vi "Decode Type Descriptor.vi"(4 "error in (no error)":errorcluster, 7 "TypeDesc":i16[](array[numeric])) -> (0 "error out":errorcluster, 1 "Type Descriptor":i16[](array[numeric]), 2 "Control Label":string, 3 "Type String":string)   [LabVIEW 2010]
doc: "In decoding the type descriptor, data types that contain other data types need to be handled differently. Specifically, these would be arrays and clusters. The generic term \"blob\" is used throughout this program to refer to these types as a whole.\n\nThe string output by this code is generally not useful to send to another VI, but it is obvious how it corresponds to the data type of the input. The purpose of the code is to see how the type descriptor is formatted and how to decode it.\n\nThe low byte of the appropriate element of the type descriptor array contains the type of the data. See small string selection case and large operate case for what data types correspond to what numbers.\n\nThe blob parameter arrays in the shift registers (size, index, element, done, dimension) are manipulated as a stack to allow decoding even deeply nested data types.\n\nGenerally, each case in the large operate case structure performs the following tasks:\n1. Uses \"Calculate String Info.vi\" and \"Replace Substring\" to assemble the type string.\n2. Uses \"Calculate Blob Info.vi\" to calculate the next type descriptor index position.\n3. Parses out the label for the control in question from the type descriptor array.\n\nThis VI is complicated in order to support nested data types such as a cluster of arrays of clusters. For more information on the format of the type descriptor, see app note 154 at ni.com, entitled \"LabVIEW Data Storage\"."
panel:
  # "Select Help»Show Context Help and move the cursor\nover the VI icon to display help for this VI."
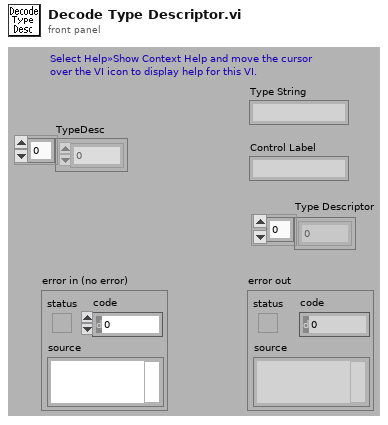
[diagram p1: front panel]
types:
  T1 = cluster{"status":bool, "code":i32, "name":string}
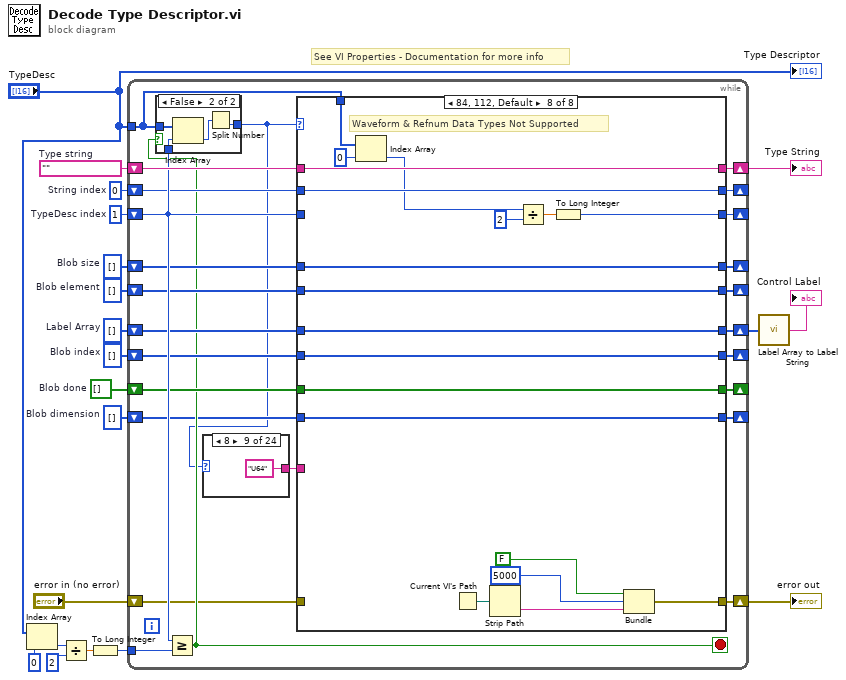
[diagram p0: block diagram]
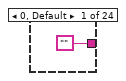
[diagram p2: hidden frame]
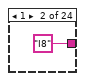
[diagram p3: hidden frame]
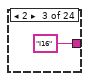
[diagram p4: hidden frame]
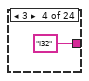
[diagram p5: hidden frame]
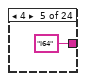
[diagram p6: hidden frame]
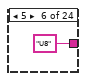
[diagram p7: hidden frame]
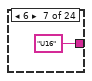
[diagram p8: hidden frame]
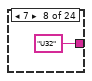
[diagram p9: hidden frame]
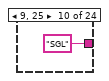
[diagram p10: hidden frame]
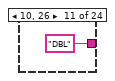
[diagram p11: hidden frame]
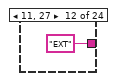
[diagram p12: hidden frame]
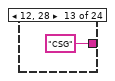
[diagram p13: hidden frame]
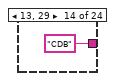
[diagram p14: hidden frame]
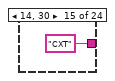
[diagram p15: hidden frame]
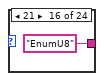
[diagram p16: hidden frame]
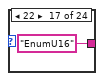
[diagram p17: hidden frame]
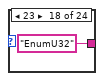
[diagram p18: hidden frame]
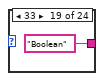
[diagram p19: hidden frame]
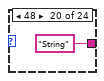
[diagram p20: hidden frame]
diagram:
  w2 = i16[] []  # Blob dimension
  w5 = i16[] []  # Blob index
  w6 = bool[] []  # Blob done
  w7 = i16[] []  # Blob element
  w8 = i16[] []  # Blob size
  w10 = i16[] []  # Label Array
  w11 = 0  # String index
  w14 = 1  # TypeDesc index
  w20 = ""  # Type string
  # "See VI Properties - Documentation for more info"
  n1 = Index Array(array="TypeDesc", index=0) -> (element=w18:i16)
  n2 = Divide(x=w18, y=i16 2) -> (x/y=w16:dbl)
  n3 = To Long Integer(number=w16) -> (32bit integer=w15:i32)
  n4 = while {
    shift-left: w2 -> [w23]
    shift-right: [w22] -> _
    shift-left: "error in (no error)" -> [w25]
    shift-right: [w24] -> w4
    shift-left: w5 -> [w30]
    shift-right: [w29] -> _
    shift-left: w6 -> [w32]
    shift-right: [w31] -> _
    shift-left: w10 -> [w34]
    shift-right: [w35] -> w9
    shift-left: w7 -> [w37]
    shift-right: [w36] -> _
    shift-left: w8 -> [w39]
    shift-right: [w38] -> _
    shift-left: w11 -> [w41]
    shift-right: [w40] -> _
    shift-left: w14 -> [w42]
    shift-right: [w45] -> _
    tunnel: w15 -> [w27]
    shift-left: w20 -> [w44]
    shift-right: [w43] -> w12
    tunnel: "TypeDesc" -> [w33]
    stop <- w28 stop-if-true
    n5 = Greater Or Equal?(x=w42, y=w27) -> (x >= y?=w28:bool)
    n6 = case shown="False" w28 {
      tunnel: w33 -> [_ w74]
      tunnel: [u8 0 w72] -> w21
      tunnel: w42 -> [_ w71]
      frame True {
      }
      frame False {
        n7 = Index Array(array=w74, index=w71) -> (element=w73:i16)
        n8 = Split Number(x=w73) -> (lo(x)=w72:u8)  [unwired: 1 out]
      }
    }
    n9 = case shown="8" w21 {
      tunnel: ["" "I8" ("string") "I16" ("string") "I32" ("string") "I64" ("string") "U8" ("string") "U16" ("string") "U32" ("string") "U64" ("string") "SGL" ("string") "DBL" ("string") "EXT" ("string") "CSG" ("string") "CDB" ("string") "CXT" ("string") "EnumU8" ("string") "EnumU16" ("string") "EnumU32" ("string") "Boolean" ("string") "String" ("string") "Path" ("string") "Pict" ("string") "ArrayD()" ("string") "Cluster()" ("string")] -> w26
      frame 0, Default {
      }
      frame 1 {
      }
      frame 2 {
      }
      frame 3 {
      }
      frame 4 {
      }
      frame 5 {
      }
      frame 6 {
      }
      frame 7 {
      }
      frame 8 {
      }
      frame 9, 25 {
      }
      frame 10, 26 {
      }
      frame 11, 27 {
      }
      frame 12, 28 {
      }
      frame 13, 29 {
      }
      frame 14, 30 {
      }
      frame 21 {
      }
      frame 22 {
      }
      frame 23 {
      }
      frame 33 {
      }
      frame 48 {
      }
      frame 50 {
      }
      frame 51 {
      }
      frame 64 {
      }
      frame 80 {
      }
    }
    n10 = case shown="84, 112, Default" w21 {
      tunnel: [w77 w97 w140 w186 w217 w247 w358 w450] -> w45
      tunnel: w42 -> [w77 w89 w130 w176 w209 w252 w363 _]
      tunnel: [w84 w106 w148 w195 w226 w255 w366 w462] -> w43
      tunnel: w44 -> [w84 w107 w149 w196 w227 w256 w367 w462]
      tunnel: [w80 w108 w116 w197 w228 w243 w354 w458] -> w35
      tunnel: w41 -> [w83 w95 w138 w184 w215 w254 w365 w461]
      tunnel: [w83 w91 w134 w180 w211 w253 w364 w461] -> w40
      tunnel: [w82 w101 w143 w190 w221 w248 w359 w460] -> w38
      tunnel: w39 -> [w82 w94 w137 w183 w214 w251 w362 w460]
      tunnel: [w81 w102 w144 w191 w222 w249 w360 w459] -> w36
      tunnel: w37 -> [w81 w93 w136 w182 w213 w250 w361 w459]
      tunnel: w34 -> [w80 _ _ _ _ _ _ w458]
      tunnel: w33 -> [_ w90 w121 w177 w210 w239 w350 w455]
      tunnel: w32 -> [w79 w104 w146 w193 w224 w242 w353 w456]
      tunnel: [w79 w103 w145 w192 w223 w246 w357 w456] -> w31
      tunnel: w30 -> [w78 w99 w142 w188 w219 w245 w356 w457]
      tunnel: [w78 w98 w141 w187 w218 w244 w355 w457] -> w29
      tunnel: w26 -> [_ w87 w132 w179 w207 w238 w349 _]
      tunnel: w25 -> [w76 w86 w131 w178 w204 w237 w348 _]
      tunnel: [w76 w86 w131 w178 w204 w237 w348 w445] -> w24
      tunnel: [w75 w85 w115 w167 w203 w235 w346 w444] -> w22
      tunnel: w23 -> [w75 w85 w115 w167 w203 w236 w347 w444]
      frame 0 {
        # "No-op, finished"
      }
      frame 1..14, 33 {
        # "Scalar Numeric & Boolean Data Types"
        n11 = Decrement(x=w89) -> (x-1=w88:i32)
        n12 = call "Calculate String Info.vi"("Str in"=w87, "Str idx in"=w95, "Blob size in"=w94, "Blob elem in"=w93, "Is scalar"=TRUE) -> ("Str out"=w92:string, "Str idx out"=w91:i32)  [unwired: 9 out]
        n13 = Index Array(array=w90, index=w88) -> (element=w100:i16)
        n14 = call "Calculate Blob Info.vi"("TypeDesc idx in"=w89, "Sub-desc size"=w100, "Blob size in"=w94, "Blob elem in"=w93, "Blob idx in"=w99, "Blob done in"=w104, "Blob dim"=w85) -> ("TypeDesc idx out"=w97:i32, "Blob size out"=w101:i16[], "Blob elem out"=w102:i16[], "Blob idx out"=w98:i16[], "Blob done out"=w103:bool[])  [unwired: 4 out]
        n15 = Divide(x=w100, y=i16 2) -> (x/y=w113:dbl)
        n16 = Replace Substring(2:0 ("length (len. of substring)"), 3:w95, 4:w92, 5:w107) -> (1:w106:string)  [unwired: 1 out]
        n17 = To Long Integer(number=w113) -> (32bit integer=w112:i32)
        n18 = Increment(x=w89) -> (x+1=w114:i32)
        n19 = Subtract(x=w112, y=2) -> (x-y=w109:i32)
        n20 = Array Subset(array=w90, index=w114, length=w109) -> (w108:i16[])
      }
      frame 21..23 {
        # "Enumerated Integer Data Types"
        n21 = Increment(x=w130) -> (x+1=w127:i32)
        n22 = Decrement(x=w130) -> (x-1=w133:i32)
        n23 = call "Calculate String Info.vi"("Str in"=w132, "Str idx in"=w138, "Blob size in"=w137, "Blob elem in"=w136, "Is scalar"=TRUE) -> ("Str out"=w135:string, "Str idx out"=w134:i32)  [unwired: 9 out]
        n24 = Index Array(array=w121, index=w133) -> (element=w120:i16)
        n25 = Index Array(array=w121, index=w127) -> (element=w129:i16)
        n26 = Increment(x=w127) -> (x+1=w126:i32)
        n27 = call "Calculate Blob Info.vi"("TypeDesc idx in"=w130, "Sub-desc size"=w120, "Blob size in"=w137, "Blob elem in"=w136, "Blob idx in"=w142, "Blob done in"=w146, "Blob dim"=w115) -> ("TypeDesc idx out"=w140:i32, "Blob size out"=w143:i16[], "Blob elem out"=w144:i16[], "Blob idx out"=w141:i16[], "Blob done out"=w145:bool[])  [unwired: 4 out]
        n28 = To Long Integer(number=w129) -> (32bit integer=w128:i32)
        n29 = for {
          N: w128 -> [_]
          shift-right: [w150] -> w123
          shift-left: w126 -> [w155]
          tunnel: w121 -> [w166]
          shift-right: [w159] -> w124
          shift-left: TRUE -> [w156]
          n30 = Index Array(array=w166, index=w155) -> (element=w165:i16)
          n31 = Split Number(x=w165) -> (hi(x)=w164:u8, lo(x)=w163:u8)
          n32 = Select(t=w164, s=w156, f=w163) -> (s? t:f=w158:u8)
          n33 = Quotient & Remainder(x=w158, y=u8 2) -> (x-y*floor(x/y)=w161:u8, floor(x/y)=w160:u8)
          n34 = To Long Integer(number=w160) -> (32bit integer=w154:i32)
          n35 = Equal To 0?(x=w161) -> (x = 0?=w157:bool)
          n36 = And(x=w156, y=w157) -> (x .and. y?=w153:bool)
          n37 = Add(x=w154, y=w155) -> (x+y=w152:i32)
          n38 = Increment(x=w152) -> (x+1=w151:i32)
          n39 = Exclusive Or(1:w156, 2:w157) -> (0:w159:bool)
          n40 = Select(t=w152, s=w153, f=w151) -> (s? t:f=w150:i32)
        }
        n41 = Increment(x=w123) -> (x+1=w122:i32)
        n42 = To Long Integer(number=w120) -> (32bit integer=w118:i32)
        n43 = Select(t=w123, s=w124, f=w122) -> (s? t:f=w119:i32)
        n44 = Subtract(x=w118, y=w119) -> (x-y=w117:i32)
        n45 = Array Subset(array=w121, index=w119, length=w117) -> (w116:i16[])
        n46 = Replace Substring(2:0 ("length (len. of substring)"), 3:w138, 4:w135, 5:w149) -> (1:w148:string)  [unwired: 1 out]
      }
      frame 25..30 {
        # "Physical Quantity Scalar Numeric Data Types"
        n47 = Decrement(x=w176) -> (x-1=w169:i32)
        n48 = call "Calculate String Info.vi"("Str in"=w179, "Str idx in"=w184, "Blob size in"=w183, "Blob elem in"=w182, "Is scalar"=TRUE) -> ("Str out"=w181:string, "Str idx out"=w180:i32)  [unwired: 9 out]
        n49 = Increment(x=w176) -> (x+1=w175:i32)
        n50 = Index Array(array=w177, index=w175) -> (element=w174:i16)
        n51 = Index Array(array=w177, index=w169) -> (element=w189:i16)
        n52 = call "Calculate Blob Info.vi"("TypeDesc idx in"=w176, "Sub-desc size"=w189, "Blob size in"=w183, "Blob elem in"=w182, "Blob idx in"=w188, "Blob done in"=w193, "Blob dim"=w167) -> ("TypeDesc idx out"=w186:i32, "Blob size out"=w190:i16[], "Blob elem out"=w191:i16[], "Blob idx out"=w187:i16[], "Blob done out"=w192:bool[])  [unwired: 4 out]
        n53 = Multiply(x=w174, y=i16 2) -> (x*y=w172:i16)
        n54 = Divide(x=w189, y=i16 2) -> (x/y=w201:dbl)
        n55 = Add(x=w172, y=i16 3) -> (x+y=w170:i16)
        n56 = Replace Substring(2:0 ("length (len. of substring)"), 3:w184, 4:w181, 5:w196) -> (1:w195:string)  [unwired: 1 out]
        n57 = To Long Integer(number=w201) -> (32bit integer=w200:i32)
        n58 = To Long Integer(number=w170) -> (32bit integer=w168:i32)
        n59 = Add(x=w168, y=w169) -> (x+y=w202:i32)
        n60 = Subtract(x=w200, y=w168) -> (x-y=w198:i32)
        n61 = Array Subset(array=w177, index=w202, length=w198) -> (w197:i16[])
      }
      frame 48, 50, 51 {
        # "String, Path, & Pict Data Types"
        n62 = Decrement(x=w209) -> (x-1=w208:i32)
        n63 = call "Calculate String Info.vi"("Str in"=w207, "Str idx in"=w215, "Blob size in"=w214, "Blob elem in"=w213, "Is scalar"=TRUE) -> ("Str out"=w212:string, "Str idx out"=w211:i32)  [unwired: 9 out]
        n64 = Index Array(array=w210, index=w208) -> (element=w220:i16)
        n65 = call "Calculate Blob Info.vi"("TypeDesc idx in"=w209, "Sub-desc size"=w220, "Blob size in"=w214, "Blob elem in"=w213, "Blob idx in"=w219, "Blob done in"=w224, "Blob dim"=w203) -> ("TypeDesc idx out"=w217:i32, "Blob size out"=w221:i16[], "Blob elem out"=w222:i16[], "Blob idx out"=w218:i16[], "Blob done out"=w223:bool[])  [unwired: 4 out]
        n66 = Divide(x=w220, y=i16 2) -> (x/y=w233:dbl)
        n67 = Increment(x=w209) -> (x+1=w205:i32)
        n68 = Replace Substring(2:0 ("length (len. of substring)"), 3:w215, 4:w212, 5:w227) -> (1:w226:string)  [unwired: 1 out]
        n69 = To Long Integer(number=w233) -> (32bit integer=w232:i32)
        n70 = Increment(x=w205) -> (x+1=w206:i32)
        n71 = Increment(x=w206) -> (x+1=w234:i32)
        n72 = Subtract(x=w232, y=4) -> (x-y=w229:i32)
        n73 = Array Subset(array=w210, index=w234, length=w229) -> (w228:i16[])
      }
      frame 64 {
        # "Array"
        n74 = Index Array(array=w242, index=0) -> (element=w240:bool)
        n75 = case shown="True" w240 {
          tunnel: w256 -> [w293 w342]
          tunnel: [w292 w342] -> w255
          tunnel: w254 -> [w274 w314]
          tunnel: [w277 w317] -> w253
          tunnel: w252 -> [w290 w306]
          tunnel: w251 -> [w273 w313]
          tunnel: w250 -> [w272 w340]
          tunnel: [w289 w320] -> w249
          tunnel: [w288 w321] -> w248
          tunnel: [w266 w325] -> w247
          tunnel: w242 -> [w285 w341]
          tunnel: [w283 w318] -> w246
          tunnel: w245 -> [w281 w337]
          tunnel: [w280 w319] -> w244
          tunnel: [i16[] [] w334] -> w243
          tunnel: w239 -> [w275 w310]
          tunnel: w238 -> [w263 _]
          tunnel: w236 -> [w259 w297]
          tunnel: [w258 w307] -> w235
          frame False {
            w271 = i16 1 ("new element/subarray")
            w260 = 0 ("index")
            n76 = Increment(x=w290) -> (x+1=w287:i32)
            n77 = Index Array(array=w275, index=w287) -> (element=w257:i16)
            n78 = Number To Decimal String(number=w257) -> (decimal integer string=w261:string)  [unwired: 1 out]
            n79 = Increment(x=w287) -> (x+1=w286:i32)
            n80 = Multiply(x=w257, y=i16 2) -> (x*y=w268:i16)
            n81 = Increment(x=w286) -> (x+1=w269:i32)
            n82 = To Long Integer(number=w268) -> (32bit integer=w267:i32)
            n83 = Insert Into Array(array=w273, index=w260, new element=w271) -> (w288:i16[])
            n84 = Insert Into Array(array=w272, index=w260, new element=w271) -> (w289:i16[])
            n85 = Insert Into Array(array=w281, index=w260, new element=i16 0) -> (w280:i16[])
            n86 = Insert Into Array(array=w285, index=w260, new element=FALSE ("new element/subarray")) -> (w283:bool[])
            n87 = Insert Into Array(array=w259, index=w260, new element=w257) -> (w258:i16[])
            n88 = Replace Substring(2:0 ("length (len. of substring)"), 3:5 ("offset (0)"), 4:w261, 5:w263) -> (1:w262:string)  [unwired: 1 out]
            n89 = Add(x=w267, y=w269) -> (x+y=w266:i32)
            n90 = call "Calculate String Info.vi"("Str in"=w262, "Str idx in"=w274, "Blob size in"=w273, "Blob elem in"=w272, "Is scalar"=FALSE) -> ("Str out"=w278:string, "Str idx out"=w277:i32)  [unwired: 9 out]
            n91 = Replace Substring(2:0 ("length (len. of substring)"), 3:w274, 4:w278, 5:w293) -> (1:w292:string)  [unwired: 1 out]
          }
          frame True {
            w339 = 0 ("index")
            w338 = 1 ("length")
            n92 = Decrement(x=w306) -> (x-1=w311:i32)
            n93 = Index Array(array=w310, index=w311) -> (element=w309:i16)
            n94 = Index Array(array=w337, index=0) -> (element=w329:i16)
            n95 = Delete From Array(array=w313, length=w338, index=w339) -> (array with subset deleted=w312:i16[])  [unwired: 1 out]
            n96 = Delete From Array(array=w340, length=w338, index=w339) -> (array with subset deleted=w324:i16[])  [unwired: 1 out]
            n97 = Delete From Array(array=w337, length=w338, index=w339) -> (array with subset deleted=w323:i16[])  [unwired: 1 out]
            n98 = Delete From Array(array=w341, length=w338, index=w339) -> (array with subset deleted=w322:bool[])  [unwired: 1 out]
            n99 = Subtract(x=w309, y=w329) -> (x-y=w332:i16)
            n100 = Divide(x=w329, y=i16 2) -> (x/y=w328:dbl)
            n101 = Array Size(array=w312) -> (size(s)=w316:i32)
            n102 = Divide(x=w332, y=i16 2) -> (x/y=w333:dbl)
            n103 = To Long Integer(number=w328) -> (32bit integer=w327:i32)
            n104 = Delete From Array(array=w297, length=1 ("index"), index=0 ("length")) -> (array with subset deleted=w307:i16[])  [unwired: 1 out]
            n105 = call "Calculate Blob Info.vi"("TypeDesc idx in"=w306, "Sub-desc size"=w309, "Blob size in"=w312, "Blob elem in"=w324, "Blob idx in"=w323, "Blob done in"=w322, "Blob dim"=w307) -> ("TypeDesc idx out"=w325:i32, "Blob size out"=w321:i16[], "Blob elem out"=w320:i16[], "Blob idx out"=w319:i16[], "Blob done out"=w318:bool[])  [unwired: 4 out]
            n106 = To Long Integer(number=w333) -> (32bit integer=w302:i32)
            n107 = Not Equal To 0?(x=w316) -> (x != 0?=w315:bool)
            n108 = Add(x=w327, y=2) -> (x+y=w305:i32)
            n109 = Index Array(array=w297, index=0) -> (element=w295:i16)
            n110 = case shown="True" w315 {
              tunnel: w314 -> [w343 w345]
              tunnel: [w343 w344] -> w317
              frame False {
              }
              frame True {
                n111 = Increment(x=w345) -> (x+1=w344:i32)
              }
            }
            n112 = To Long Integer(number=w295) -> (32bit integer=w300:i32)
            n113 = Multiply(x=w300, y=2) -> (x*y=w294:i32)
            n114 = Compound Arithmetic op=ADD(w306, w305, w294) -> (w304:i32)
            n115 = Compound Arithmetic op=ADD(w305, w294, 3 ("y")) -> (w301:i32)
            n116 = Subtract(x=w301, y=w302) -> (x-y=w331:i32)
            n117 = Array Subset(array=w310, index=w304, length=w331) -> (w334:i16[])
          }
        }
      }
      frame 80 {
        # "Cluster"
        n118 = Index Array(array=w353, index=0) -> (element=w351:bool)
        n119 = case shown="True" w351 {
          tunnel: w367 -> [w397 w440]
          tunnel: [w396 w440] -> w366
          tunnel: w365 -> [w376 w408]
          tunnel: [w379 w411] -> w364
          tunnel: w363 -> [w394 w398]
          tunnel: w362 -> [w375 w407]
          tunnel: w361 -> [w374 w438]
          tunnel: [w391 w414] -> w360
          tunnel: [w390 w415] -> w359
          tunnel: [w373 w419] -> w358
          tunnel: w353 -> [w387 w439]
          tunnel: [w385 w412] -> w357
          tunnel: w356 -> [w383 w435]
          tunnel: [w382 w413] -> w355
          tunnel: [i16[] [] w431] -> w354
          tunnel: w350 -> [w377 w404]
          tunnel: w349 -> [w372 _]
          tunnel: w347 -> [w371 w402]
          tunnel: [w370 w399] -> w346
          frame False {
            w369 = 0 ("index")
            n120 = Increment(x=w394) -> (x+1=w389:i32)
            n121 = Index Array(array=w377, index=w389) -> (element=w393:i16)
            n122 = Increment(x=w389) -> (x+1=w388:i32)
            n123 = Increment(x=w388) -> (x+1=w373:i32)
            n124 = Insert Into Array(array=w375, index=w369, new element=w393) -> (w390:i16[])
            n125 = Insert Into Array(array=w374, index=w369, new element=i16 1 ("new element/subarray")) -> (w391:i16[])
            n126 = Insert Into Array(array=w383, index=w369, new element=i16 0) -> (w382:i16[])
            n127 = Insert Into Array(array=w387, index=w369, new element=FALSE ("new element/subarray")) -> (w385:bool[])
            n128 = Insert Into Array(array=w371, index=w369, new element=i16 0 ("new element/subarray")) -> (w370:i16[])
            n129 = call "Calculate String Info.vi"("Str in"=w372, "Str idx in"=w376, "Blob size in"=w375, "Blob elem in"=w374, "Is scalar"=FALSE) -> ("Str out"=w380:string, "Str idx out"=w379:i32)  [unwired: 9 out]
            n130 = Replace Substring(2:0 ("length (len. of substring)"), 3:w376, 4:w380, 5:w397) -> (1:w396:string)  [unwired: 1 out]
          }
          frame True {
            w437 = 0 ("index")
            w436 = 1 ("length")
            n131 = Decrement(x=w398) -> (x-1=w405:i32)
            n132 = Index Array(array=w404, index=w405) -> (element=w403:i16)
            n133 = Index Array(array=w435, index=0) -> (element=w424:i16)
            n134 = Delete From Array(array=w407, length=w436, index=w437) -> (array with subset deleted=w406:i16[])  [unwired: 1 out]
            n135 = Delete From Array(array=w438, length=w436, index=w437) -> (array with subset deleted=w418:i16[])  [unwired: 1 out]
            n136 = Delete From Array(array=w435, length=w436, index=w437) -> (array with subset deleted=w417:i16[])  [unwired: 1 out]
            n137 = Delete From Array(array=w439, length=w436, index=w437) -> (array with subset deleted=w416:bool[])  [unwired: 1 out]
            n138 = Divide(x=w424, y=i16 2) -> (x/y=w423:dbl)
            n139 = Subtract(x=w403, y=w424) -> (x-y=w429:i16)
            n140 = Array Size(array=w406) -> (size(s)=w410:i32)
            n141 = To Long Integer(number=w423) -> (32bit integer=w422:i32)
            n142 = Divide(x=w429, y=i16 2) -> (x/y=w430:dbl)
            n143 = Delete From Array(array=w402, length=1 ("index"), index=0 ("length")) -> (array with subset deleted=w399:i16[])  [unwired: 1 out]
            n144 = call "Calculate Blob Info.vi"("TypeDesc idx in"=w398, "Sub-desc size"=w403, "Blob size in"=w406, "Blob elem in"=w418, "Blob idx in"=w417, "Blob done in"=w416, "Blob dim"=w399) -> ("TypeDesc idx out"=w419:i32, "Blob size out"=w415:i16[], "Blob elem out"=w414:i16[], "Blob idx out"=w413:i16[], "Blob done out"=w412:bool[])  [unwired: 4 out]
            n145 = Not Equal To 0?(x=w410) -> (x != 0?=w409:bool)
            n146 = To Long Integer(number=w430) -> (32bit integer=w428:i32)
            n147 = Add(x=w422, y=2) -> (x+y=w420:i32)
            n148 = Add(x=w398, y=w420) -> (x+y=w426:i32)
            n149 = case shown="True" w409 {
              tunnel: w408 -> [w441 w443]
              tunnel: [w441 w442] -> w411
              frame False {
              }
              frame True {
                n150 = Increment(x=w443) -> (x+1=w442:i32)
              }
            }
            n151 = Subtract(x=w428, y=3) -> (x-y=w427:i32)
            n152 = Array Subset(array=w404, index=w426, length=w427) -> (w431:i16[])
          }
        }
      }
      frame 84, 112, Default {
        # "Waveform & Refnum Data Types Not Supported"
        n153 = Index Array(array=w455, index=0) -> (element=w453:i16)
        n154 = Current VI's Path() -> (path=w449:path)
        n155 = Strip Path(path=w449) -> (name=w446:string)  [unwired: 1 out]
        n156 = Divide(x=w453, y=i16 2) -> (x/y=w451:dbl)
        n157 = To Long Integer(number=w451) -> (32bit integer=w450:i32)
        n158 = Bundle("status"=FALSE, "code"=5000, "name"=w446) -> (w445:T1)  [unwired: 1 out]
      }
    }
  }
  "Type String" <- w12
  "error out" <- w4
  n159 = call "Label Array to Label String.vi"("Label Array"=w9) -> ("Label String"=→"Control Label":string)
  "Type Descriptor" <- "TypeDesc"
